vi "formatEvtTelDetails.vi"(7 "functionEnum":enum16{"event", "telemetry"}(ring), 8 "error in (no error)":errorcluster, 9 "name":string="move", 10 "detailsString":string, 11 "TcpServer.lvclass":refnum<class "TcpServer.lvclass">) -> (0 "error out":errorcluster, 2 "jsonString":string, 3 "TcpServer.lvclass":refnum<class "TcpServer.lvclass">)   [LabVIEW 2018, in "TcpServer.lvclass"]
doc: "Convert the event or the telemetry message into a JSON format. You can choose if is event or telemetry with the function enum provided. If name control is empty, an error message will be created to inform other processes about this error."
uses:
  TcpServer.lvclass
  <vilib>/Utility/error.llb/Error Cluster From Error Code.vi
  <vilib>/ErrorRing/Error Ring.xnode
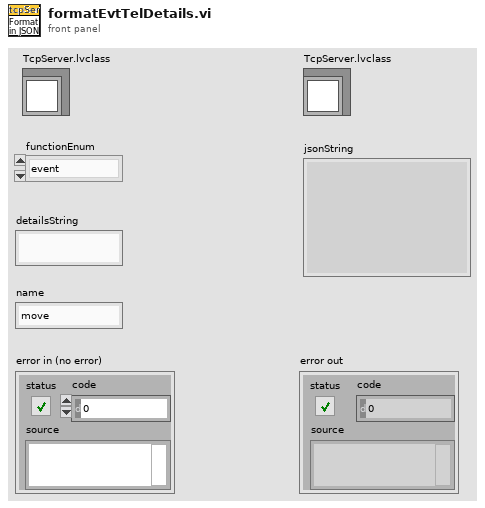
[diagram p1: front panel]
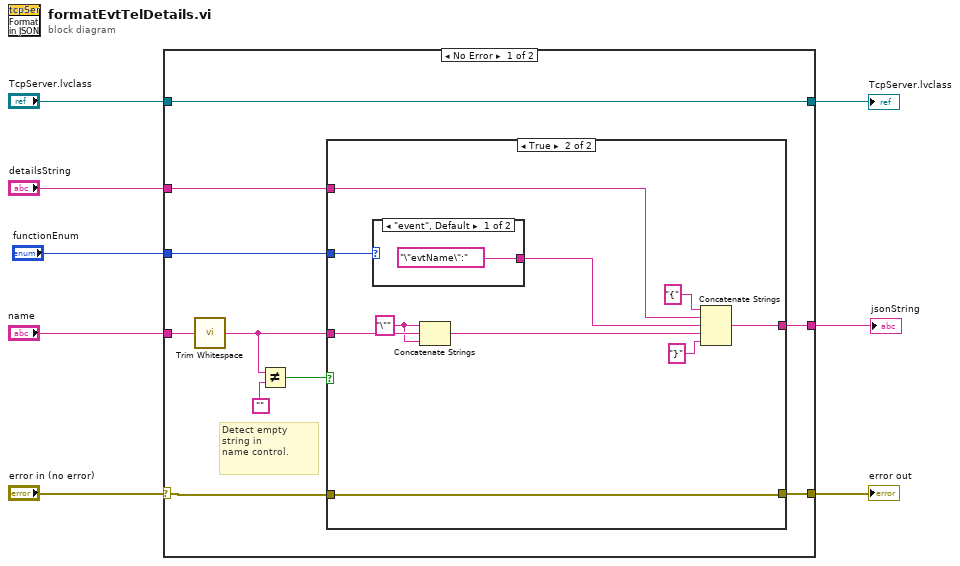
[diagram p0: block diagram]
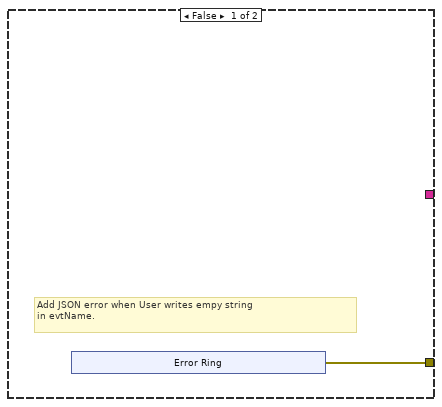
[diagram p2: hidden frame]
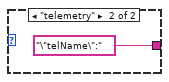
[diagram p3: hidden frame]
diagram:
  n1 = case shown="No Error" "error in (no error)" {
    selector: "error in (no error)" -> [w12 w36]
    tunnel: [w18 _] -> w3
    tunnel: "detailsString" -> [w17 _]
    tunnel: "name" -> [w14 _]
    tunnel: "TcpServer.lvclass" -> [w16 w37]
    tunnel: [w16 w37] -> w5
    tunnel: [w11 w36] -> w4
    tunnel: "functionEnum" -> [w10 _]
    frame No Error {
      # "Detect empty\nstring in \nname control."
      n2 = call <vilib>:"Trim Whitespace.vi"("string"=w14) -> ("trimmed string"=w9:string)  [unwired: 1 in]
      n3 = Not Equal?(x=w9, y="") -> (x != y?=w13:bool)
      n4 = case shown="True" w13 {
        tunnel: [_ w33] -> w18
        tunnel: w17 -> [_ w26]
        tunnel: w9 -> [_ w32]
        tunnel: w12 -> [_ w28]
        tunnel: [w19 w28] -> w11
        tunnel: w10 -> [_ w27]
        frame False {
          # "Add JSON error when User writes empy string\nin evtName."
          n5 = xnode "Error Ring"() -> ("error out"=w19:errorcluster)
        }
        frame True {
          w29 = "\"" ("string")
          n6 = case shown="\"event\", Default" w27 {
            tunnel: ["\"evtName\":" "\"telName\":"] -> w25
            frame "event", Default {
            }
            frame "telemetry" {
            }
          }
          n7 = Concatenate Strings(w29, w32, w29) -> (w24:string)
          n8 = Concatenate Strings("{" ("string"), w26, w25, w24, "}" ("string")) -> (w33:string)
        }
      }
    }
    frame Error {
    }
  }
  "jsonString" <- w3
  "error out" <- w4
  "TcpServer.lvclass" <- w5
